vi "FxParabola.vi"(6 "偏移":dbl, 7 "采样频率":dbl=200.0, 8 "平移":dbl, 9 "倍率":dbl, 10 "终点时间":dbl, 11 "起点时间":dbl) -> (0 "Y":dbl[](array[numeric]), 3 "X":dbl[](array[numeric]))   [LabVIEW 2020, in "Curve Editor.lvlib"]
uses:
  Curve Editor.lvlib
panel:
  out "XY图":cluster{dbl[], dbl[]}(graph)
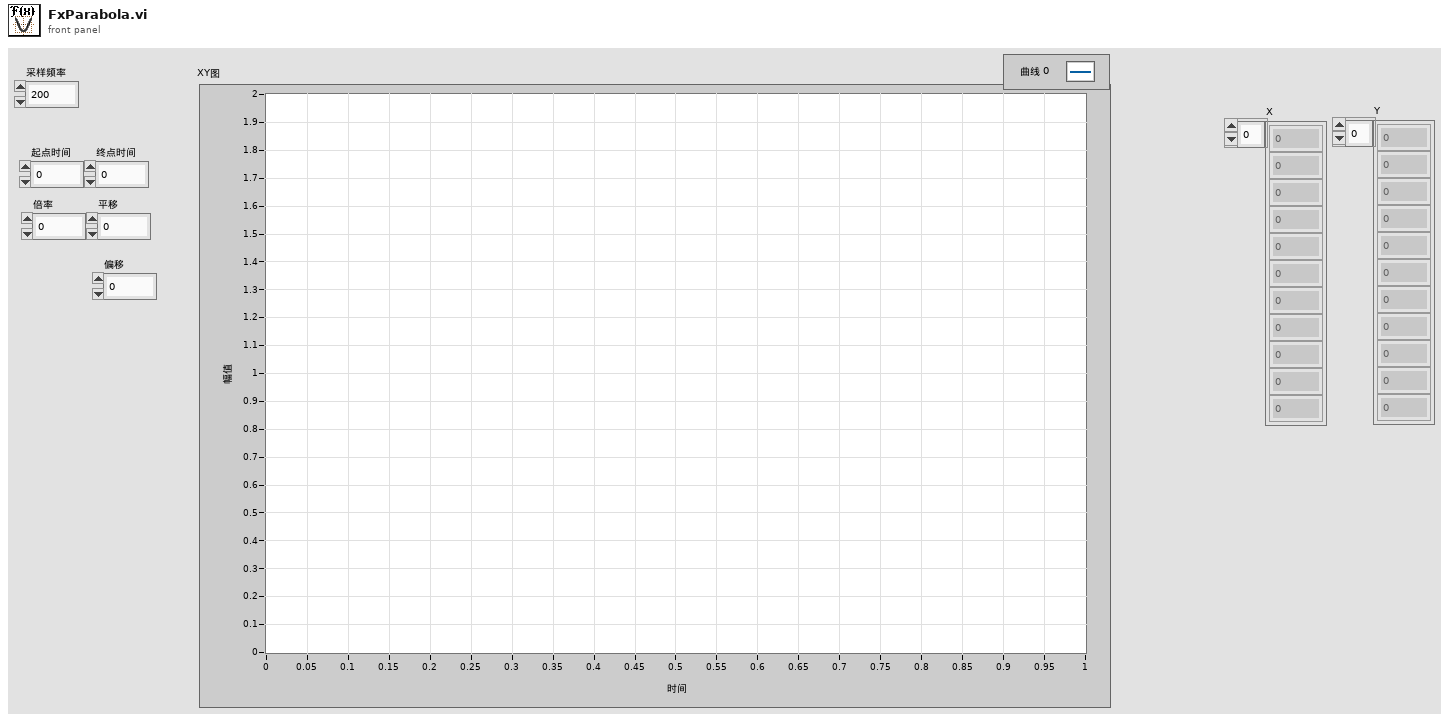
[diagram p1: front panel]
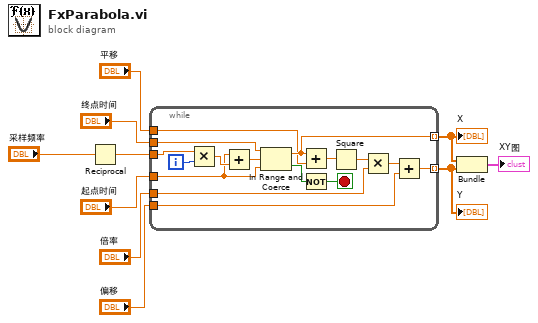
[diagram p0: block diagram]
diagram:
  n1 = Reciprocal(x="采样频率") -> (1/x=w9:dbl)
  n2 = while {
    tunnel: [w18] -> w10 mode=indexing
    tunnel: "起点时间" -> [w19]
    tunnel: "终点时间" -> [w26]
    tunnel: w9 -> [w24]
    tunnel: "平移" -> [w17]
    tunnel: "倍率" -> [w14]
    tunnel: "偏移" -> [w12]
    tunnel: [w11] -> w3 mode=indexing
    i -> [w25]
    stop <- w21 stop-if-true
    n3 = Multiply(x=w24, y=w25) -> (x*y=w20:dbl)
    n4 = Add(x=w19, y=w20) -> (x+y=w23:dbl)
    n5 = In Range and Coerce(upper limit=w26, x=w23, lower limit=w19) -> (coerced(x)=w18:dbl, In Range?=w22:bool)
    n6 = Add(x=w18, y=w17) -> (x+y=w16:dbl)
    n7 = Not(x=w22) -> (.not. x?=w21:bool)
    n8 = Square(x=w16) -> (x^2=w15:dbl)
    n9 = Multiply(x=w15, y=w14) -> (x*y=w13:dbl)
    n10 = Add(x=w13, y=w12) -> (x+y=w11:dbl)
  }
  "X" <- w10
  "Y" <- w3
  n11 = Bundle(w10, w3) -> (→"XY图":cluster{dbl[], dbl[]})  [unwired: 1 in]
